vi "download_archive.vi"(8 "error in (no error)":errorcluster, 10 "target_path":path, 11 "path":string) -> (0 "error out":errorcluster)   [LabVIEW 2015, in "lv-dropbox.lvlib" / "v2.lvlib"]
uses:
  v2.lvlib
  private/_controls/content_type.ctl
  private/_subvis/advanced/parse_header-single.vi
  <vilib>/httpClient/POSTBuffer.vi
  lv-dropbox.lvlib
  <vilib>/httpClient/LabVIEWHTTPClient.lvlib
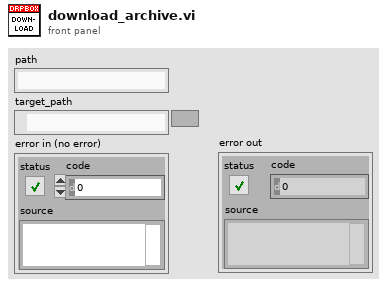
[diagram p1: front panel]
types:
  T1 = typedef "lv-dropbox.lvlib/content_type.ctl" = enum16{"<content_type>", "application/json", "application/octet-stream", "application/x-www-form-urlencoded"}
  T2 = cluster{"name":string, "path_lower":string, "id":string, "client_modified":string, "server_modified":string, "rev":string, "size":u64}
  T3 = enum16{"open", "replace", "create", "open or create", "replace or create", "replace or create with confirmation"}
  T4 = typedef "LabVIEWHTTPClient.lvlib/ClientHandle.ctl" = refnum<k1>
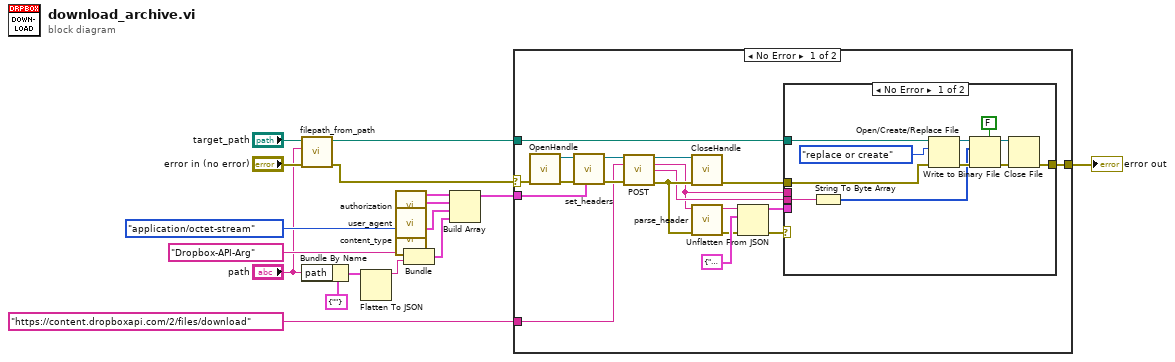
[diagram p0: block diagram]
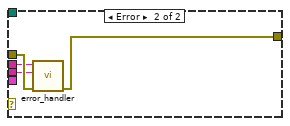
[diagram p2: hidden frame]
diagram:
  n1 = call "filepath_from_path.vi"("error in (no error)"="error in (no error)", "path"="path", "filepath in"="target_path") -> ("error out"=w3:errorcluster, "filepath out"=w5:path)  [unwired: 7 in]
  n2 = Bundle By Name(cluster=cluster{"path":string} {"path"=""}, "path"="path") -> (w9:cluster{"path":string})
  n3 = Flatten To JSON(anything=w9) -> (JSON string=w8:string)  [unwired: 2 in, 1 out]
  n4 = call "authorization.vi"() -> ("header"=w16:cluster{"header":string, "value":string})  [unwired: 11 in]
  n5 = call "user_agent.vi"() -> ("header"=w15:cluster{"header":string, "value":string})  [unwired: 11 in]
  n6 = call "content_type.vi"("content_type"=content_type."application/octet-stream") -> ("header"=w17:cluster{"header":string, "value":string})  [unwired: 10 in]
  n7 = Bundle("header"="Dropbox-API-Arg", "JSON string"=w8) -> (w2:cluster{"header":string, "JSON string":string})  [unwired: 1 in]
  n8 = Build Array(w16, w15, w17, w2) -> (w13:cluster{"header":string, "JSON string":string}[])
  n9 = case shown="No Error" w3 {
    selector: w3 -> [w30 w52]
    tunnel: w13 -> [w22 _]
    tunnel: "https://content.dropboxapi.com/2/files/download" ("url") -> [w29 _]
    tunnel: [w27 w52] -> w11
    tunnel: w5 -> [w26 _]
    frame No Error {
      n10 = call <vilib>:"OpenHandle.vi"("error in (no error)"=w30) -> ("client handle out"=w33:T4, "error out"=w23:errorcluster)  [unwired: 13 in]
      n11 = call "set_headers.vi"("header_value []"=w22, "error in (no error)"=w23, "client_handle in"=w33) -> ("error out"=w31:errorcluster, "client_handle out"=w32:T4)  [unwired: 7 in]
      n12 = call-poly <vilib>:"POST.vi"("client handle"=w32, "url"=w29, "error in (no error)"=w31) -> ("client handle out"=w35:T4, "headers"=w18:string, "body"=w28:string, "error out"=w36:errorcluster)  [unwired: 9 in]
      n13 = call <vilib>:"CloseHandle.vi"("client handle"=w35, "error in (no error)"=w36) -> ("error out"=w20:errorcluster)  [unwired: 13 in]
      n14 = call-poly "parse_header.vi"("error in (no error)"=w36, "headers"=w18) -> ("error out"=w24:errorcluster, "value"=w25:string)  [unwired: 8 in]
      n15 = Unflatten From JSON(JSON string=w25, type and defaults=T2 {"name"="", "path_lower"="", "id"="", "client_modified"="", "server_modified"="", "rev"="", "size"=0}, error in (no error)=w24) -> (value=w19:T2, error out=w21:errorcluster)  [unwired: 4 in]
      n16 = case shown="No Error" w21 {
        tunnel: w28 -> [w43 w48]
        tunnel: [w39 w50] -> w27
        tunnel: w26 -> [w38 _]
        tunnel: w20 -> [w37 w51]
        tunnel: w19 -> [_ _]
        tunnel: w18 -> [_ w49]
        frame No Error {
          n17 = String To Byte Array(string=w43) -> (unsigned byte array=w41:u8[])
          n18 = Open/Create/Replace File(file path (use dialog)=w38, error in=w37, operation (0:open)=T3."replace or create") -> (refnum out=w47:refnum<file>, error out=w44:errorcluster)  [unwired: 3 in, 1 out]
          n19 = Write to Binary File(file (use dialog)=w47, data=w41, error in=w44, 5:FALSE ("prepend array or string size? (T)")) -> (refnum out=w46:refnum<file>, error out=w45:errorcluster)  [unwired: 2 in, 1 out]
          n20 = Close File(refnum=w46, error in=w45) -> (error out=w39:errorcluster)  [unwired: 1 out]
        }
        frame Error {
          n21 = call "error_handler.vi"("error in (no error)"=w51, "body"=w48, "headers"=w49) -> ("error out"=w50:errorcluster)  [unwired: 8 in]
        }
      }
    }
    frame Error {
    }
  }
  "error out" <- w11
